vi "niScope Set External Clock.vi"(8 "error in":errorcluster, 9 "clock source":T1=enum."VAL_CLK_IN", 10 "ref. clock rate [Hz] (0: use internal clock)":dbl format="%#_13p", 11 "niScope reference in":refnum<k15>) -> (0 "error out":errorcluster, 1 "Reference Clock Rate Out":dbl, 2 "PLL Lock Status":bool, 3 "reference out":refnum<k15>, 5 "Reference Clock Source Out":string)   [LabVIEW 2013, in "niScope Virtual Digitizer.lvlib"]
doc: "Sets the clock source and clock rate for NI Scope and reads them to verify correct setting. For internal clock use 0 Hz frequency (default)."
uses:
  niScope Virtual Digitizer.lvlib
  niScope Reference Clock.ctl
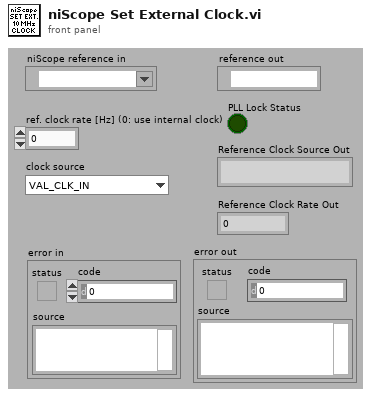
[diagram p1: front panel]
types:
  T1 = typedef "niScope Virtual Digitizer.lvlib/niScope Reference Clock.ctl" = enum16{"VAL_NO_SOURCE", "VAL_CLK_IN", "VAL_PXI_CLOCK", "VAL_EXTERNAL"}
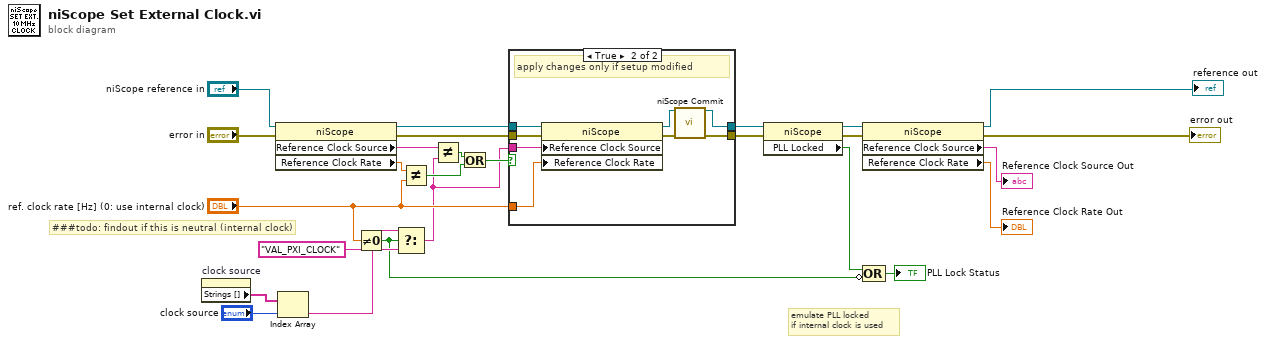
[diagram p0: block diagram]
diagram:
  # "###todo: findout if this is neutral (internal clock)"
  # "emulate PLL locked\nif internal clock is used"
  n1 = property on="clock source" class="Enum (strict)"() -> ("Strings []"=w3:string[])  [unwired: 2 in, 2 out]
  n2 = property class="niScope"(reference="niScope reference in", error in="error in") -> (reference out=w11:refnum<k15>, error out=w16:errorcluster, "Reference Clock Source"=w8:string, "Reference Clock Rate"=w15:dbl)
  n3 = Index Array(array=w3, index="clock source") -> (element=w1:string)
  n4 = Not Equal To 0?(x="ref. clock rate [Hz] (0: use internal clock)") -> (x != 0?=w4:bool)
  n5 = Select(t=w1, s=w4, f="VAL_PXI_CLOCK" ("Clocking:Reference (Input) Clock Source")) -> (s? t:f=w7:string)
  n6 = Not Equal?(x=w15, y="ref. clock rate [Hz] (0: use internal clock)") -> (x != y?=w13:bool)
  n7 = Not Equal?(x=w8, y=w7) -> (x != y?=w14:bool)
  n8 = Or(x=w14, y=w13) -> (x .or. y?=w12:bool)
  n9 = case shown="True" w12 {
    tunnel: [w27 w34] -> w18
    tunnel: [w28 w33] -> w17
    tunnel: w11 -> [w27 w32]
    tunnel: w16 -> [w28 w31]
    tunnel: "ref. clock rate [Hz] (0: use internal clock)" -> [_ w30]
    tunnel: w7 -> [_ w29]
    frame False {
    }
    frame True {
      # "apply changes only if setup modified"
      n10 = property class="niScope"(reference=w32, error in=w31, "Reference Clock Source"=w29, "Reference Clock Rate"=w30) -> (reference out=w36:refnum<k15>, error out=w35:errorcluster)
      n11 = call <instrlib>:"niScope Commit.vi"("instrument handle"=w36, "error in"=w35) -> ("instrument handle out"=w34:refnum<k15>, "error out"=w33:errorcluster)  [unwired: 12 in]
    }
  }
  n12 = property class="niScope"(reference=w18, error in=w17) -> (reference out=w22:refnum<k15>, error out=w21:errorcluster, "PLL Locked"=w5:bool)
  n13 = property class="niScope"(reference=w22, error in=w21) -> (reference out=→"reference out":refnum<k15>, error out=→"error out":errorcluster, "Reference Clock Source"=→"Reference Clock Source Out":string, "Reference Clock Rate"=→"Reference Clock Rate Out":dbl)
  n14 = Compound Arithmetic op=OR(w5, invert w4) -> (→"PLL Lock Status":bool)
